vi "LINC Write Telemetry.vi"(4 "raw byte offset (default)":i32=-1, 5 "data names":string[](array[string]), 6 "raw data":string, 7 "packet name":string, 8 "error in (no error)":errorcluster, 9 "options":T1, 10 "packet":variant, 11 "LINC session":refnum<class "LINC.lvclass">) -> (0 "error out":errorcluster, 3 "dup LINC session":refnum<class "LINC.lvclass">)   [LabVIEW 2018, in "STEPkgDriver_LINC.lvlib" / "LINC.lvclass"]
uses:
  LINC.lvclass
  STEPkgDriver_LINC.lvlib
  LINC Global Mode.ctl
  LINC Global Session Mode.ctl
  LINC Global Config Mode.ctl
  LINC Port Config.ctl
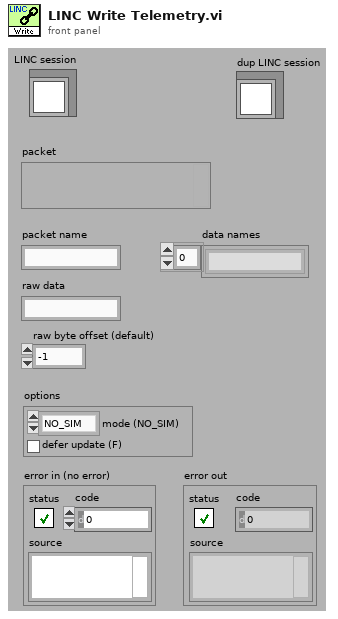
[diagram p1: front panel]
types:
  T1 = cluster{"mode (NO_SIM)":enum16{"NO_SIM", "SIM_EN", "SIM_DS"}, "defer update (F)":bool}
  T2 = typedef "STEPkgDriver_LINC.lvlib/LINC Global Config Mode.ctl" = enum16{"INIT", "CLEAR", "SET_CMD_CB", "SET_TLM_CB", "SET_CMD_FIELDS", "SET_TLM_FIELDS", "SET_ID", "GET_CONFIG"}
  T3 = typedef "STEPkgDriver_LINC.lvlib/LINC Global Mode.ctl" = enum16{"INIT", "CLEAR", "ADD_PKT_HDR", "ADD_PKT", "GET_PKT_NAMES", "GET_PKT_DESC", "GET_PKT_HDR", "GET_PKT", "SET_PKT", "SET_DATA", "SIM_EN", "SIM_DS"}
  T4 = typedef "STEPkgDriver_LINC.lvlib/LINC Global Session Mode.ctl" = enum16{"INIT", "CLEAR", "ADD_SESSION", "SET_CONNECTION", "SET_LISTENER", "SET_REFERENCE", "GET_SESSION"}
  T5 = typedef "STEPkgDriver_LINC.lvlib/LINC Port Config.ctl" = enum16{"ALL", "CMD_ALL", "TLM_ALL", "TLM_BASIC"}
  T6 = typedef "STEPkgDriver_LINC.lvlib/LINC Format Prototype.ctl" = cluster{"type":string, "bit offset":i32, "bit size":i32, "format":string, "unit":string, "description":string, "state values":i64[], "states":string[], "max":string, "min":string, "default":string, "array":bool, "bit element size":i32, "poly bound":dbl[], "poly scale":cluster{"coefficients":dbl[]}[], "labview size":i32, "simulate":bool, "ID":bool, "required":bool}
  T7 = typedef "STEPkgDriver_LINC.lvlib/LINC Sim Ops.ctl" = cluster{"byte":i32, "mask":u8}
  T8 = typedef "STEPkgDriver_LINC.lvlib/LINC Config.ctl" = cluster{"cmd callback":refnum<vi>, "tlm callback":refnum<vi>, "cmd ID bitoffset":i32, "cmd ID bitsize":i32, "cmd IDs":i32[], "tlm ID bitoffset":i32, "tlm ID bitsize":i32, "tlm IDs":i32[], "cmd header fields":i32, "tlm header fields":i32, "tlm header size":i32}
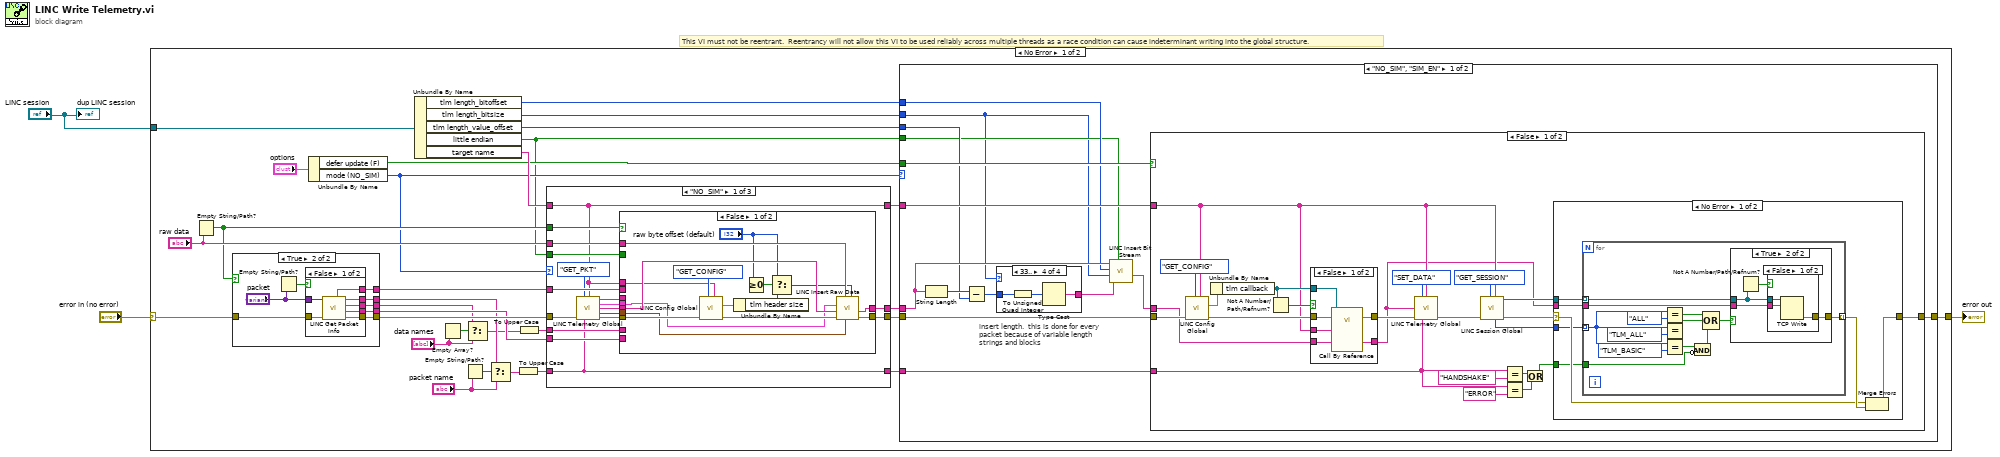
[diagram p0: block diagram]
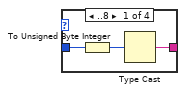
[diagram p2: hidden frame]
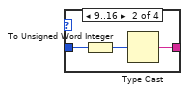
[diagram p3: hidden frame]
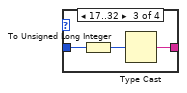
[diagram p4: hidden frame]
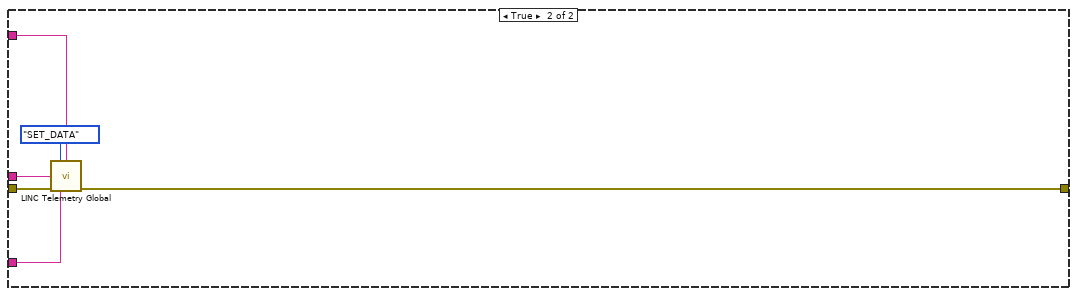
[diagram p9: hidden frame]
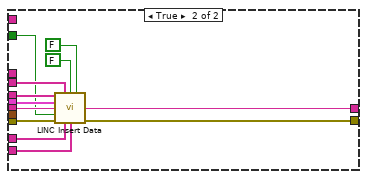
[diagram p11: hidden frame]
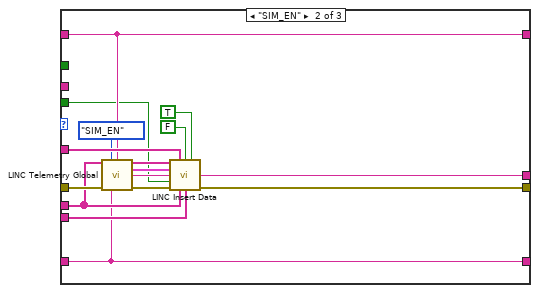
[diagram p12: hidden frame]
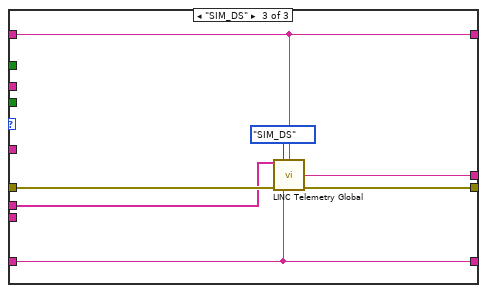
[diagram p13: hidden frame]
diagram:
  # "This VI must not be reentrant.  Reentrancy will not allow this VI to be used reliably across multiple threads as a race condition can cause indeterminant writing into the global structure."
  n1 = case shown="No Error" "error in (no error)" {
    selector: "error in (no error)" -> [w7 w210]
    tunnel: [w33 w210] -> w3
    tunnel: "LINC session" -> [w6 _]
    frame No Error {
      n2 = Empty String/Path?(string/path="raw data") -> (empty?=w26:bool)
      n3 = case shown="True" w26 {
        tunnel: w7 -> [w193 w201]
        tunnel: [w193 w200] -> w30
        tunnel: [_ w199] -> w24
        tunnel: [_ w198] -> w20
        tunnel: [_ w197] -> w29
        tunnel: [_ w196] -> w28
        frame False {
        }
        frame True {
          n4 = Empty String/Path?(string/path="packet") -> (empty?=w194:bool)
          n5 = case shown="False" w194 {
            tunnel: w201 -> [w208 w209]
            tunnel: [w207 w209] -> w200
            tunnel: [w206 _] -> w199
            tunnel: [w205 _] -> w198
            tunnel: [w204 _] -> w197
            tunnel: [w203 _] -> w196
            tunnel: "packet" -> [w202 _]
            frame False {
              n6 = call "LINC Get Packet Info.vi"("error in (no error)"=w208, "packet"=w202) -> ("error out"=w207:errorcluster, "member data"=w204:string[], "member names"=w205:string[], "packet name"=w206:string, "member types"=w203:string[])  [unwired: 5 in]
            }
            frame True {
            }
          }
        }
      }
      n7 = Unbundle By Name("options") -> ("defer update (F)"=w16:bool, "mode (NO_SIM)"=w9:enum16{"NO_SIM", "SIM_EN", "SIM_DS"})
      n8 = Unbundle By Name(w6) -> ("tlm length_bitoffset"=w13:i32, "tlm length_bitsize"=w12:i32, "tlm length_value_offset"=w11:i32, "little endian"=w8:bool, "target name"=w31:string)
      n9 = Empty Array?(array="data names") -> (empty?=w21:bool)
      n10 = Empty String/Path?(string/path="packet name") -> (empty?=w25:bool)
      n11 = Select(t=w20, s=w21, f="data names") -> (s? t:f=w18:string[])
      n12 = Select(t=w24, s=w25, f="packet name") -> (s? t:f=w10:string)
      n13 = To Upper Case(1:w10) -> (0:w5:string)
      n14 = To Upper Case(1:w18) -> (0:w4:string[])
      n15 = case shown="\"NO_SIM\"" w9 {
        tunnel: [w131 w174 w188] -> w32
        tunnel: w31 -> [w127 w173 w189]
        tunnel: w5 -> [w129 w171 w186]
        tunnel: w30 -> [w142 w185 w192]
        tunnel: w29 -> [w141 w184 _]
        tunnel: [w130 w172 w187] -> w14
        tunnel: w28 -> [w136 w179 _]
        tunnel: "raw data" -> [w135 _ _]
        tunnel: w26 -> [w134 _ _]
        tunnel: w4 -> [w133 w175 w190]
        tunnel: [w127 w173 w189] -> w22
        tunnel: [w129 w171 w186] -> w15
        tunnel: w8 -> [w128 w170 _]
        frame "NO_SIM" {
          n16 = call "LINC Telemetry Global.vi"("mode"=LINC_Global_Mode."GET_PKT", "target name"=w127, "error in (no error)"=w142, "packet name"=w129) -> ("values out"=w139:string[], "item formats out"=w138:T6[], "data out"=w137:string, "sim ops"=w126:T7[], "error out"=w140:errorcluster)  [unwired: 7 in]
          n17 = case shown="False" w134 {
            tunnel: w133 -> [_ w169]
            tunnel: w141 -> [_ w168]
            tunnel: w140 -> [w153 w167]
            tunnel: [w157 w166] -> w131
            tunnel: w139 -> [_ w165]
            tunnel: w138 -> [w143 w164]
            tunnel: w137 -> [w151 w163]
            tunnel: [w155 w162] -> w130
            tunnel: w136 -> [_ w160]
            tunnel: w135 -> [w156 _]
            tunnel: w128 -> [_ w158]
            tunnel: w127 -> [w145 _]
            tunnel: w126 -> [w144 _]
            frame False {
              n18 = call "LINC Config Global.vi"("target name"=w145, "mode"=LINC_Global_Config_Mode."GET_CONFIG", "error in (no error)"=w153) -> ("error out"=w152:errorcluster, "config out"=w148:T8)  [unwired: 7 in]
              n19 = Unbundle By Name(w148) -> ("tlm header size"=w147:i32)
              n20 = Greater Or Equal To 0?(x="raw byte offset (default)") -> (x >= 0?=w150:bool)
              n21 = Select(t="raw byte offset (default)", s=w150, f=w147) -> (s? t:f=w146:i32)
              n22 = call "LINC Insert Raw Data.vi"("raw byte offset (0)"=w146, "sim ops"=w144, "raw data"=w156, "error in (no error)"=w152, "data in"=w151, "item formats in"=w143) -> ("error out"=w157:errorcluster, "data out"=w155:string)  [unwired: 4 in]
            }
            frame True {
              n23 = call "LINC Insert Data.vi"("item names"=w165, "member types"=w160, "scale"=FALSE, "simulate"=FALSE, "item formats"=w164, "data in"=w163, "little endian"=w158, "error in (no error)"=w167, "member names"=w169, "member data"=w168) -> ("data out"=w162:string, "error out"=w166:errorcluster)  [unwired: 4 in]
            }
          }
        }
        frame "SIM_EN" {
          n24 = call "LINC Telemetry Global.vi"("item names in"=w175, "mode"=LINC_Global_Mode."SIM_EN", "target name"=w173, "error in (no error)"=w185, "packet name"=w171) -> ("values out"=w182:string[], "item formats out"=w181:T6[], "data out"=w180:string, "error out"=w183:errorcluster)  [unwired: 6 in, 1 out]
          n25 = call "LINC Insert Data.vi"("item names"=w182, "member types"=w179, "scale"=FALSE, "simulate"=TRUE, "item formats"=w181, "data in"=w180, "little endian"=w170, "error in (no error)"=w183, "member names"=w175, "member data"=w184) -> ("data out"=w172:string, "error out"=w174:errorcluster)  [unwired: 4 in]
        }
        frame "SIM_DS" {
          n26 = call "LINC Telemetry Global.vi"("item names in"=w190, "mode"=LINC_Global_Mode."SIM_DS", "target name"=w189, "error in (no error)"=w192, "packet name"=w186) -> ("data out"=w187:string, "error out"=w188:errorcluster)  [unwired: 6 in, 3 out]
        }
      }
      n27 = case shown="\"NO_SIM\", \"SIM_EN\"" w9 {
        tunnel: [w47 w125] -> w33
        tunnel: w32 -> [w46 w125]
        tunnel: w22 -> [w45 _]
        tunnel: w16 -> [w44 _]
        tunnel: w15 -> [w43 _]
        tunnel: w14 -> [w41 _]
        tunnel: w13 -> [w40 _]
        tunnel: w12 -> [w34 _]
        tunnel: w11 -> [w38 _]
        tunnel: w8 -> [w37 _]
        frame "NO_SIM", "SIM_EN" {
          # "insert length.  this is done for every packet because of variable length strings and blocks"
          n28 = String Length(string=w41) -> (length=w39:i32)
          n29 = Subtract(x=w39, y=w38) -> (x-y=w36:i32)
          n30 = case shown="33.." w34 {
            tunnel: w36 -> [w49 w52 w55 w58]
            tunnel: [w48 w51 w54 w57] -> w35
            frame ..8 {
              n31 = To Unsigned Byte Integer(number=w49) -> (unsigned 8bit integer=w50:u8)
              n32 = Type Cast(x=w50) -> (*(type *) &x=w48:string)  [unwired: 1 in]
            }
            frame 9..16 {
              n33 = To Unsigned Word Integer(number=w52) -> (unsigned 16bit integer=w53:u16)
              n34 = Type Cast(x=w53) -> (*(type *) &x=w51:string)  [unwired: 1 in]
            }
            frame 17..32 {
              n35 = To Unsigned Long Integer(number=w55) -> (unsigned 32bit integer=w56:u32)
              n36 = Type Cast(x=w56) -> (*(type *) &x=w54:string)  [unwired: 1 in]
            }
            frame 33.. {
              n37 = To Unsigned Quad Integer(1:w58) -> (0:w59:u64)
              n38 = Type Cast(x=w59) -> (*(type *) &x=w57:string)  [unwired: 1 in]
            }
          }
          n39 = call "LINC Insert Bit Stream.vi"("little endian"=w37, "data to insert"=w35, "bit size"=w34, "bit offset"=w40, "data in"=w41) -> ("data out"=w42:string)  [unwired: 4 in]
          n40 = case shown="False" w44 {
            tunnel: [w68 w122] -> w47
            tunnel: w46 -> [w73 w123]
            tunnel: w42 -> [w72 w120]
            tunnel: w45 -> [w71 w121]
            tunnel: w43 -> [w63 w119]
            frame False {
              n41 = call "LINC Config Global.vi"("target name"=w71, "mode"=LINC_Global_Config_Mode."GET_CONFIG", "error in (no error)"=w73) -> ("error out"=w76:errorcluster, "config out"=w78:T8)  [unwired: 7 in]
              n42 = Unbundle By Name(w78) -> ("tlm callback"=w79:refnum<vi>)
              n43 = Not A Number/Path/Refnum?(number/path/refnum=w79) -> (NaN/Path/Refnum?=w80:bool)
              n44 = case shown="False" w80 {
                tunnel: [w116 w118] -> w75
                tunnel: w72 -> [w115 w117]
                tunnel: [w114 w117] -> w69
                tunnel: w76 -> [w113 w118]
                tunnel: w79 -> [w112 _]
                tunnel: w71 -> [w111 _]
                frame False {
                  n45 = call-by-ref "?"(reference=w112, error in=w113, "command in"=w115, "target name"=w111) -> (error out=w116:errorcluster, "command out"=w114:string)  [unwired: 2 out]
                }
                frame True {
                }
              }
              n46 = call "LINC Telemetry Global.vi"("mode"=LINC_Global_Mode."SET_DATA", "target name"=w71, "data in"=w69, "error in (no error)"=w75, "packet name"=w63) -> ("error out"=w70:errorcluster)  [unwired: 6 in, 4 out]
              n47 = call "LINC Session Global.vi"("target name"=w71, "mode"=LINC_Global_Session_Mode."GET_SESSION", "error in (no error)"=w70) -> ("error out"=w67:errorcluster, "connections out"=w81:refnum<k5>[], "port config"=w66:T5[])  [unwired: 4 in, 2 out]
              n48 = Equal?(x=w63, y="HANDSHAKE") -> (x = y?=w62:bool)
              n49 = Equal?(x=w63, y="ERROR") -> (x = y?=w61:bool)
              n50 = Or(x=w62, y=w61) -> (x .or. y?=w60:bool)
              n51 = case shown="No Error" w67 {
                selector: w67 -> [w85 w110]
                tunnel: w81 -> [w89 _]
                tunnel: w69 -> [w88 _]
                tunnel: [w86 w110] -> w68
                tunnel: w66 -> [w84 _]
                tunnel: w60 -> [w83 _]
                frame No Error {
                  n52 = for {
                    tunnel: w88 -> [w102]
                    tunnel: w89 -> [w101] mode=indexing
                    tunnel: [w100] -> w87 mode=indexing
                    tunnel: w84 -> [w96] mode=indexing
                    tunnel: w83 -> [w92]
                    n53 = Equal?(x=w96, y=LINC_Port_Config."ALL") -> (x = y?=w95:bool)
                    n54 = Equal?(x=w96, y=LINC_Port_Config."TLM_ALL") -> (x = y?=w94:bool)
                    n55 = Equal?(x=w96, y=LINC_Port_Config."TLM_BASIC") -> (x = y?=w93:bool)
                    n56 = Compound Arithmetic op=AND(w93, invert w92) -> (w91:bool)
                    n57 = Compound Arithmetic op=OR(w95, w94, w91) -> (w90:bool)
                    n58 = case shown="True" w90 {
                      tunnel: w102 -> [_ w106]
                      tunnel: w101 -> [_ w105]
                      tunnel: [_ w104] -> w100
                      frame False {
                      }
                      frame True {
                        n59 = Not A Number/Path/Refnum?(number/path/refnum=w105) -> (NaN/Path/Refnum?=w103:bool)
                        n60 = case shown="False" w103 {
                          tunnel: w106 -> [w109 _]
                          tunnel: w105 -> [w108 _]
                          tunnel: [w107 _] -> w104
                          frame False {
                            n61 = TCP Write(connection ID=w108, data in=w109) -> (error out=w107:errorcluster)  [unwired: 1 in, 3 out]
                          }
                          frame True {
                          }
                        }
                      }
                    }
                  }
                  n62 = Merge Errors(w85, w87) -> (w86:errorcluster)
                }
                frame Error {
                }
              }
            }
            frame True {
              n63 = call "LINC Telemetry Global.vi"("mode"=LINC_Global_Mode."SET_DATA", "target name"=w121, "data in"=w120, "error in (no error)"=w123, "packet name"=w119) -> ("error out"=w122:errorcluster)  [unwired: 6 in, 4 out]
            }
          }
        }
        frame "SIM_DS" {
        }
      }
    }
    frame Error {
    }
  }
  "error out" <- w3
  "dup LINC session" <- "LINC session"
